vi "Meas Result Get Access.vi"(7 "timout [s] (30s)":dbl=30.0 format="%#_13g", 8 "error in":errorcluster, 11 "results ref":refnum<vi>) -> (0 "error out":errorcluster, 3 "results data":T1)   [LabVIEW 2020]
doc: "Gets exclusive access to the result. No other process can get access until the release result is called."
uses:
  Meas Results.ctl
  bridge/Bridge Frequency Readings Data.ctl
  drivers/TWM client/Meas Proc QWTB Spectrum Data.ctl
  drivers/TWM client/TWM Phase Info.ctl
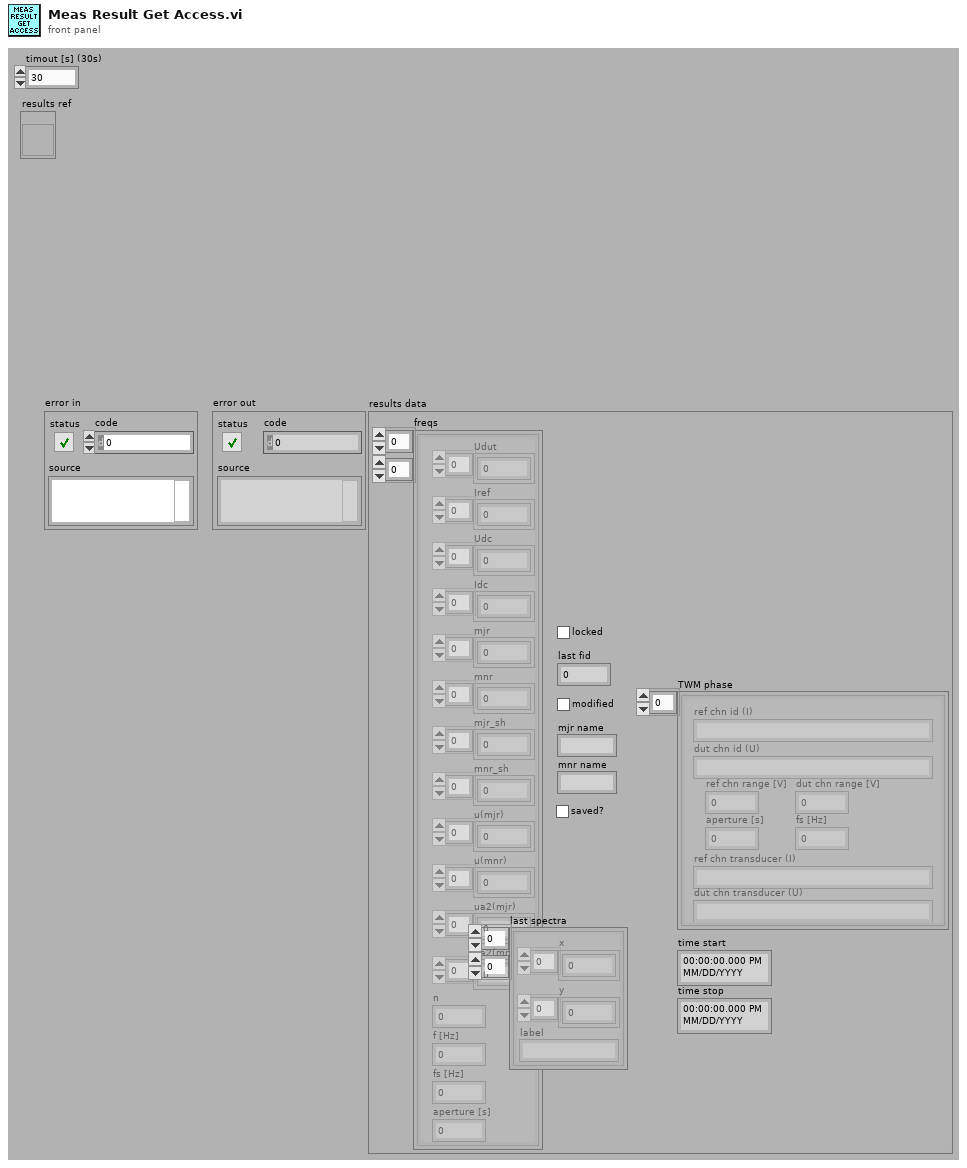
[diagram p1: front panel]
types:
  T1 = typedef "Meas Results.ctl" = cluster{"freqs":T2[][], "locked":bool, "last fid":i32, "modified":bool, "mjr name":string, "mnr name":string, "last spectra":T3[][], "saved?":bool, "TWM phase":T4[], "time start":timestamp, "time stop":timestamp}
  T2 = typedef "Bridge Frequency Readings Data.ctl" = cluster{"Udut":dbl[], "Iref":dbl[], "Udc":dbl[], "Idc":dbl[], "mjr":dbl[], "mnr":dbl[], "mjr_sh":dbl[], "mnr_sh":dbl[], "u(mjr)":dbl[], "u(mnr)":dbl[], "ua2(mjr)":dbl[], "ua2(mnr)":dbl[], "n":i32, "f [Hz]":dbl, "fs [Hz]":dbl, "aperture [s]":dbl}
  T3 = typedef "Meas Proc QWTB Spectrum Data.ctl" = cluster{"x":sgl[], "y":sgl[], "label":string}
  T4 = typedef "TWM Phase Info.ctl" = cluster{"ref chn id (I)":string, "dut chn id (U)":string, "ref chn range [V]":dbl, "dut chn range [V]":dbl, "aperture [s]":dbl, "fs [Hz]":dbl, "ref chn transducer (I)":string, "dut chn transducer (U)":string}
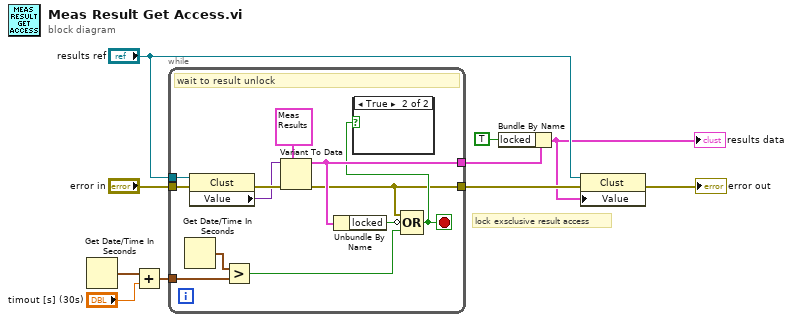
[diagram p0: block diagram]
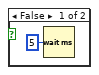
[diagram p2: hidden frame]
diagram:
  # "lock exsclusive result access"
  n1 = Get Date/Time In Seconds() -> (seconds since 1Jan1904=w7:timestamp)
  n2 = Add(x=w7, y="timout [s] (30s)") -> (x+y=w5:timestamp)
  n3 = while {
    tunnel: "results ref" -> [w22]
    tunnel: "error in" -> [w21]
    tunnel: [w11] -> w4
    tunnel: [w17] -> w8
    tunnel: w5 -> [w14]
    stop <- w12 stop-if-true
    # "wait to result unlock"
    n4 = Get Date/Time In Seconds() -> (seconds since 1Jan1904=w15:timestamp)
    n5 = property class="Clust"(reference=w22, error in=w21) -> (error out=w20:errorcluster, "Value"=w19:variant)  [unwired: 1 out]
    n6 = Greater?(x=w15, y=w14) -> (0:w13:bool)
    n7 = Variant To Data(error in=w20, type=T1 {"freqs"=[], "locked"=FALSE, "last fid"=0, "modified"=FALSE, "mjr name"="", "mnr name"="", "last spectra"=[], "saved?"=FALSE, "TWM phase"=[], "time start"=timestamp(0 s since 1904-01-01), "time stop"=timestamp(0 s since 1904-01-01)} ("Cluster"), Variant=w19) -> (data=w17:T1, error out=w11:errorcluster)
    n8 = Unbundle By Name(w17) -> ("locked"=w16:bool)
    n9 = Compound Arithmetic op=OR(w11, invert w16, w13) -> (w12:bool)
    n10 = case shown="True" w12 {
      frame False {
        n11 = Wait (ms)(milliseconds to wait=u32 5) -> ()  [unwired: 1 out]
      }
      frame True {
      }
    }
  }
  n12 = Bundle By Name(cluster=w8, "locked"=TRUE) -> (w1:T1)
  "results data" <- w1
  n13 = property class="Clust"(reference="results ref", error in=w4, "Value"=w1) -> (error out=→"error out":errorcluster)  [unwired: 1 out]
